vi "Pinout.vi"(3 "Akcja":T3, 4 "Wybór komory":T2) -> (2 "Wyjœcie":T1={"LEWO"=7, "PRAWO"=11, "GÓRA"=35, "Dӣ"=36, "CZUJNIK"=12, "I2C ADRES"=12})   [LabVIEW 2014]
uses:
  AkcjaGFV.ctl
  wykonajRuchVIs/parametryKomorVIs/WyborKomory.ctl
  pinoutVIs/PinoutLista.ctl
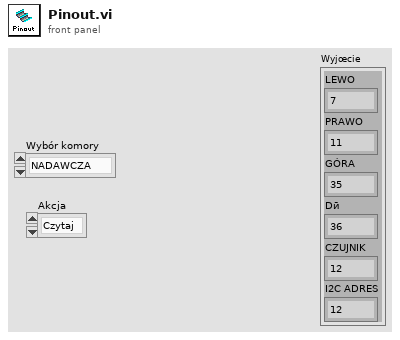
[diagram p1: front panel]
types:
  T1 = typedef "PinoutLista.ctl" = cluster{"LEWO":u8, "PRAWO":u8, "GÓRA":u8, "Dӣ":u8, "CZUJNIK":u8, "I2C ADRES":u8}
  T2 = typedef "WyborKomory.ctl" = enum16{"NADAWCZA", "ODBIORCZA"}
  T3 = typedef "AkcjaGFV.ctl" = enum16{"Czytaj", "Zapisz", "Reset"}
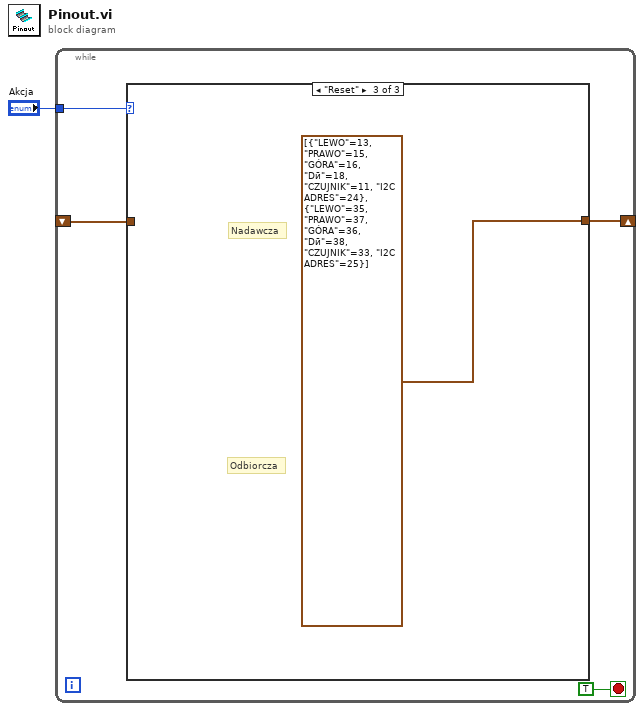
[diagram p0: block diagram]
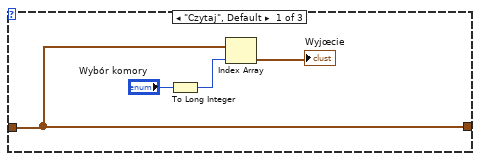
[diagram p2: hidden frame]
diagram:
  n1 = while {
    tunnel: "Akcja" -> [w4]
    shift-right: [w3] -> _
    shift-left: _ -> [w2]
    stop <- TRUE stop-if-true
    n2 = case shown="\"Reset\"" w4 {
      tunnel: [w9 w10 T1[] [{"LEWO"=13, "PRAWO"=15, "GÓRA"=16, "Dӣ"=18, "CZUJNIK"=11, "I2C ADRES"=24}, {"LEWO"=35, "PRAWO"=37, "GÓRA"=36, "Dӣ"=38, "CZUJNIK"=33, "I2C ADRES"=25}]] -> w3
      tunnel: w2 -> [w9 w10 _]
      frame "Czytaj", Default {
        n3 = To Long Integer(number="Wybór komory") -> (32bit integer=w6:i32)
        n4 = Index Array(array=w9, index=w6) -> (element=→"Wyjœcie":T1)
      }
      frame "Zapisz" {
      }
      frame "Reset" {
        # "Odbiorcza"
        # "Nadawcza"
      }
    }
  }
